vi "Read IPS Level.vi"(8 "error in (no error)":errorcluster, 11 "Instrument.Oxford1820 in":refnum<class "Instrument.Oxford1820.lvclass">) -> (0 "error out":errorcluster, 1 "N2 Level (%)":dbl, 2 "He Level (%)":dbl, 3 "Instrument.Oxford1820 out":refnum<class "Instrument.Oxford1820.lvclass">, 4 "Fill Mode":T1="ON")   [LabVIEW 2019, in "Instrument.Oxford1820.lvclass"]
uses:
  Instrument.Oxford1820.lvclass
  Typedefs/Fill Mode-Combo.ctl
  Instrument.Oxford1820.lvclass/Instrument.Oxford1820.ctl
  <instrlib>/Mercury iXX/Public/Libraries/Level Meter/Open/Open Level Meter Device.vi
  <instrlib>/Mercury iXX/Public/Libraries/Level Meter/Signals/Read/Probe Level Helium (Read).vi
  <instrlib>/Mercury iXX/Public/Libraries/Level Meter/Signals/Read/Probe Level Nitrogen (Read).vi
  <instrlib>/Mercury iXX/Public/Libraries/Level Meter/Configuration/Read/Helium Pulse Slow-Fast (Read).vi
  <instrlib>/Mercury iXX/Mercury iXX.lvlib
  <instrlib>/Mercury iXX/Public/Libraries/Level Meter.lvlib
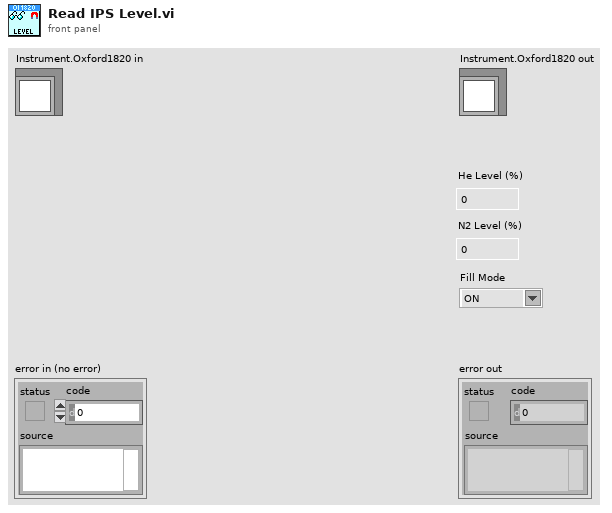
[diagram p1: front panel]
types:
  T1 = typedef "Instrument.Oxford1820.lvclass/Fill Mode-Combo.ctl" = string
  T2 = typedef "Mercury iXX.lvlib/Mercury Reference.ctl" = cluster{"Comms":refnum<visa-resource-name>, "Device ID":string[], "Comms Layer":T3, "Command":string, "Query reference":T4}
  T3 = typedef "Mercury iXX.lvlib/Comms Transport Layer.ctl" = enum16{"Ethernet TCP/IP", "USB", "ISOBus - RS-232", "GPIB"}
  T4 = typedef "Mercury iXX.lvlib/Query Dynamic Reference.ctl" = refnum<vi>
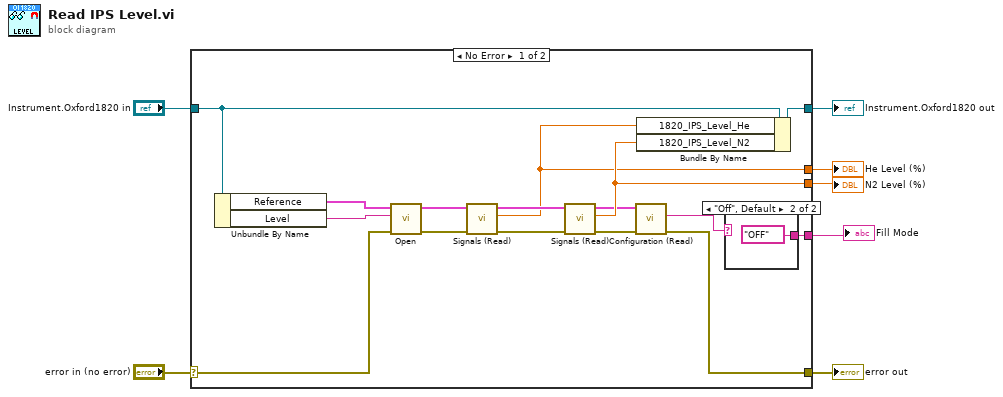
[diagram p0: block diagram]
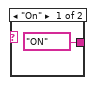
[diagram p2: hidden frame]
diagram:
  n1 = case shown="No Error" "error in (no error)" {
    selector: "error in (no error)" -> [w19 w27]
    tunnel: [w10 w27] -> w6
    tunnel: [w16 w26] -> w4
    tunnel: "Instrument.Oxford1820 in" -> [w15 w26]
    tunnel: [w13 _] -> w3
    tunnel: [w14 _] -> w2
    tunnel: [w8 _] -> w1
    frame No Error {
      n2 = Unbundle By Name(w15) -> ("Reference"=w20:T2, "Level"=w21:string)
      n3 = call-poly <instrlib>:"Open.vi"("error in (no error)"=w19, "Device Identifier"=w21, "Mercury Reference In"=w20) -> ("error out"=w23:errorcluster, "Mercury Reference Out"=w22:T2)  [unwired: 7 out]
      n4 = call-poly <instrlib>:"Signals (Read).vi"("error in"=w23, "Mercury Reference In"=w22) -> ("error out"=w18:errorcluster, "Level"=w13:dbl, "Mercury Reference Out"=w17:T2)  [unwired: 1 in, 6 out]
      n5 = call-poly <instrlib>:"Signals (Read).vi"("error in"=w18, "Mercury Reference In"=w17) -> ("error out"=w11:errorcluster, "Level"=w14:dbl, "Mercury Reference Out"=w12:T2)  [unwired: 1 in, 6 out]
      n6 = call-poly <instrlib>:"Configuration (Read).vi"("error in"=w11, "Mercury Reference In"=w12) -> ("error out"=w10:errorcluster, "Response"=w9:string)  [unwired: 6 in, 2 out]
      n7 = Bundle By Name(cluster=w15, "1820_IPS_Level_He"=w13, "1820_IPS_Level_N2"=w14) -> (w16:refnum<class "Instrument.Oxford1820.lvclass">)
      n8 = case shown="\"Off\", Default" w9 {
        tunnel: [T1 "ON" ("Fill Mode") T1 "OFF" ("Fill Mode")] -> w8
        frame "On" {
        }
        frame "Off", Default {
        }
      }
    }
    frame Error {
    }
  }
  "error out" <- w6
  "Instrument.Oxford1820 out" <- w4
  "He Level (%)" <- w3
  "N2 Level (%)" <- w2
  "Fill Mode" <- w1
